vi "Injection Command Plot.vi"(6 "Plot Selector (T=TMP, F=EPT)":bool, 9 "System":T6={"Battery [V]"=13.7, "Engine Speed [RPM]"=1000.0, "Rotations"=1, "Injector Configuration"={"Resistance [Ohm]"=1.0, "Inductance [Henery]"=0.001, "Capacitance [Farad]"=5e-06}, "Description"=""} {"Injector Configuration"."Capacitance [Farad]" format="%#_6p"; "Injector Configuration"."Inductance [Henery]" format="%#_6p"; "Injector Configuration"."Resistance [Ohm]" format="%#_6p"; "Rotations" min=1 max=2; "Engine Speed [RPM]" min=500 max=50000; "Battery [V]" min=6 max=48}, 10 "Injection Command":T1={"Mode"=enum."Off", "Digital Input"=enum."Unused", "Default Profile Index"=0, "Cal Freq [Hz]"=0.0, "Cal Duration [s]"=0.0, "Cal Increment [s]"=0.0, "Cal Pulses"=0, "TMP Command Sequence"=[{"Duration [s]"=0.0, "Level"=FALSE, "Run/Stop"=FALSE, "Profile Index"=0}, {"Duration [s]"=0.0, "Level"=FALSE, "Run/Stop"=FALSE, "Profile Index"=0}, {"Duration [s]"=0.0, "Level"=FALSE, "Run/Stop"=FALSE, "Profile Index"=0}, {"Duration [s]"=0.0, "Level"=FALSE, "Run/Stop"=FALSE, "Profile Index"=0}, {"Duration [s]"=0.0, "Level"=FALSE, "Run/Stop"=FALSE, "Profile Index"=0}, {"Duration [s]"=0.0, "Level"=FALSE, "Run/Stop"=FALSE, "Profile Index"=0}, {"Duration [s]"=0.0, "Level"=FALSE, "Run/Stop"=FALSE, "Profile Index"=0}, {"Duration [s]"=0.0, "Level"=FALSE, "Run/Stop"=FALSE, "Profile Index"=0}], "EPT TDC Offset [CAD]"=0.0, "EPT Window Start [DBTDC]"=0.0, "EPT Window End [DBTDC]"=0.0, "EPT Angles"=[{"Enable"=FALSE, "Timing [DBTDC]"=0.0, "Duration [s]"=0.0, "Profile Index"=0}, {"Enable"=FALSE, "Timing [DBTDC]"=0.0, "Duration [s]"=0.0, "Profile Index"=0}, {"Enable"=FALSE, "Timing [DBTDC]"=0.0, "Duration [s]"=0.0, "Profile Index"=0}, {"Enable"=FALSE, "Timing [DBTDC]"=0.0, "Duration [s]"=0.0, "Profile Index"=0}, {"Enable"=FALSE, "Timing [DBTDC]"=0.0, "Duration [s]"=0.0, "Profile Index"=0}, {"Enable"=FALSE, "Timing [DBTDC]"=0.0, "Duration [s]"=0.0, "Profile Index"=0}, {"Enable"=FALSE, "Timing [DBTDC]"=0.0, "Duration [s]"=0.0, "Profile Index"=0}, {"Enable"=FALSE, "Timing [DBTDC]"=0.0, "Duration [s]"=0.0, "Profile Index"=0}], "EPT Skip Fire"=FALSE, "EPT Skip Index"=0, "EPT Precharge Duration [s]"=0.0, "EPT Precharge Profile Index"=0} {"EPT Precharge Profile Index" max=15; "EPT Precharge Duration [s]" min=0 format="%#_4p"; "Default Profile Index" max=15; "Cal Increment [s]" format="%#_3p"; "TMP Command Sequence"."Profile Index" max=7; "TMP Command Sequence"."Duration [s]" min=0 max=100 format="%#_3p"; "Cal Pulses" max=511; "EPT Skip Index" max=7; "EPT Angles"."Profile Index" max=7; "EPT Angles"."Duration [s]" min=0 max=100 format="%#_3p"; "Cal Duration [s]" format="%#_3p"; "Cal Freq [Hz]" format="%#_3p"}) -> (2 "Plot":cluster{"Array":sgl[], "Array":sgl[]}[](array[cluster]))   [LabVIEW 2016, in "DCM System Explorer.lvlib"]
uses:
  DCM System Explorer.lvlib
  <vilib>/Powertrain Controls/Device Drivers/DCM/Rev0/UI/System Configuration.ctl
  <vilib>/Powertrain Controls/Device Drivers/DCM/Rev0/UI/Injector Configuration.ctl
  <vilib>/Powertrain Controls/Device Drivers/DCM/DI/RT/Command.ctl
  <vilib>/Powertrain Controls/Device Drivers/DCM/DI/FPGA/Mode.ctl
  <vilib>/Powertrain Controls/Device Drivers/DCM/Rev0/FPGA/Digital Channel.ctl
  <vilib>/Powertrain Controls/Device Drivers/DCM/DI/RT/Command Sequence.ctl
  <vilib>/Powertrain Controls/Device Drivers/DCM/DI/RT/Angle Control.ctl
  <vilib>/Powertrain Controls/Device Drivers/DCM/Rev0/UI/DCM - UI.lvlib
  <vilib>/Powertrain Controls/Device Drivers/DCM/DI/FPGA/DCM - FPGA - DI.lvlib
  <vilib>/Powertrain Controls/Device Drivers/DCM/Rev0/FPGA/DCM - FPGA.lvlib
  <vilib>/Powertrain Controls/Device Drivers/DCM/DI/RT/DCM - RT - DI.lvlib
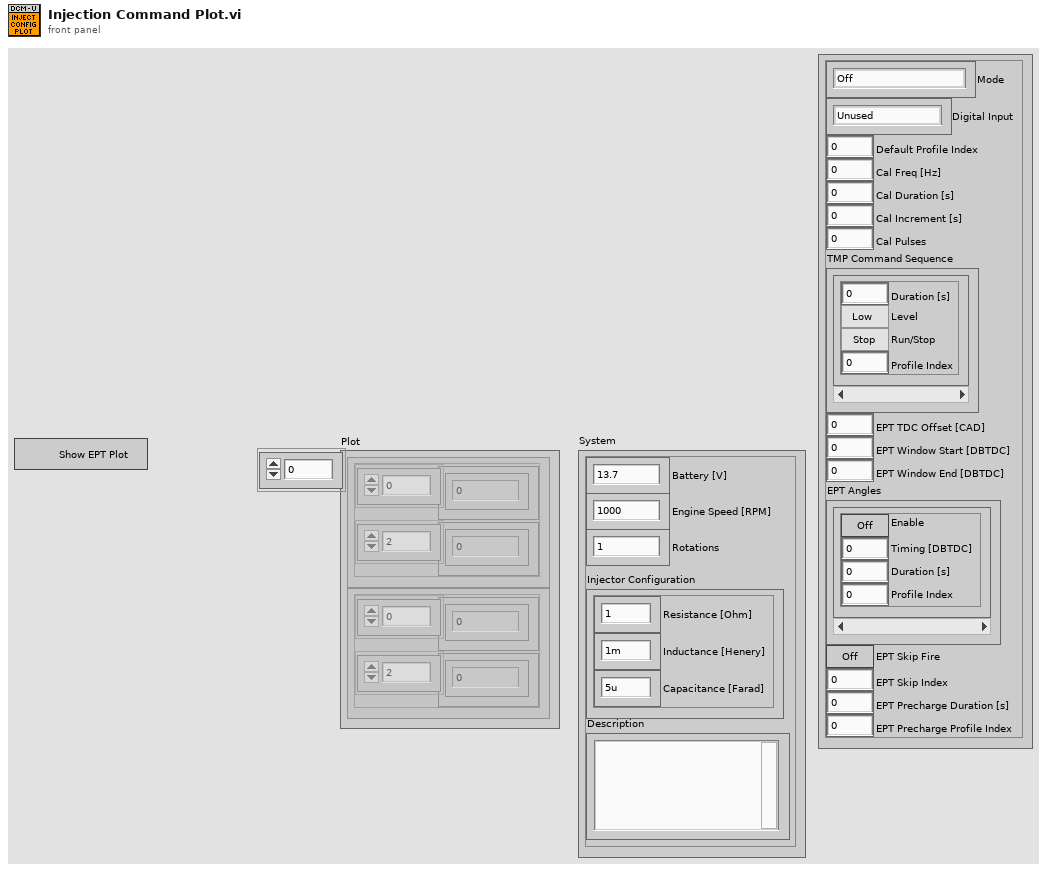
[diagram p1: front panel]
types:
  T1 = typedef "DCM - RT - DI.lvlib/Command.ctl" = cluster{"Mode":T2, "Digital Input":T3, "Default Profile Index":u8, "Cal Freq [Hz]":sgl, "Cal Duration [s]":sgl, "Cal Increment [s]":sgl, "Cal Pulses":u16, "TMP Command Sequence":T4[], "EPT TDC Offset [CAD]":sgl, "EPT Window Start [DBTDC]":sgl, "EPT Window End [DBTDC]":sgl, "EPT Angles":T5[], "EPT Skip Fire":bool, "EPT Skip Index":u8, "EPT Precharge Duration [s]":sgl, "EPT Precharge Profile Index":u8}
  T2 = typedef "DCM - FPGA - DI.lvlib/Mode.ctl" = enum8{"Off", "Direct", "Calibration", "Triggered Multi-Pulse", "Engine Position Tracking"}
  T3 = typedef "DCM - FPGA.lvlib/Digital Channel.ctl" = enum8{"Unused", "User OS", "Diff IO 1", "Diff IO 2", "Diff IO 3", "Diff IO 4", "Diff IO 5", "Diff IO 6", "Diff IO 7", "Diff IO 8", "Aux 1", "Aux 2", "Aux 3", "Aux 4", "Aux 5", "Aux 6", "Aux 7", "Aux 8", "Aux 9", "Aux 10", "Aux 11", "Aux 12", "Aux 13", "Aux 14", "Aux 15", "Aux 16"}
  T4 = typedef "DCM - RT - DI.lvlib/Command Sequence.ctl" = cluster{"Duration [s]":sgl, "Level":bool, "Run/Stop":bool, "Profile Index":u8}
  T5 = typedef "DCM - RT - DI.lvlib/Angle Control.ctl" = cluster{"Enable":bool, "Timing [DBTDC]":sgl, "Duration [s]":sgl, "Profile Index":u8}
  T6 = typedef "DCM - UI.lvlib/System Configuration.ctl" = cluster{"Battery [V]":sgl, "Engine Speed [RPM]":sgl, "Rotations":u8, "Injector Configuration":T7, "Description":string}
  T7 = typedef "DCM - UI.lvlib/Injector Configuration.ctl" = cluster{"Resistance [Ohm]":sgl, "Inductance [Henery]":sgl, "Capacitance [Farad]":sgl}
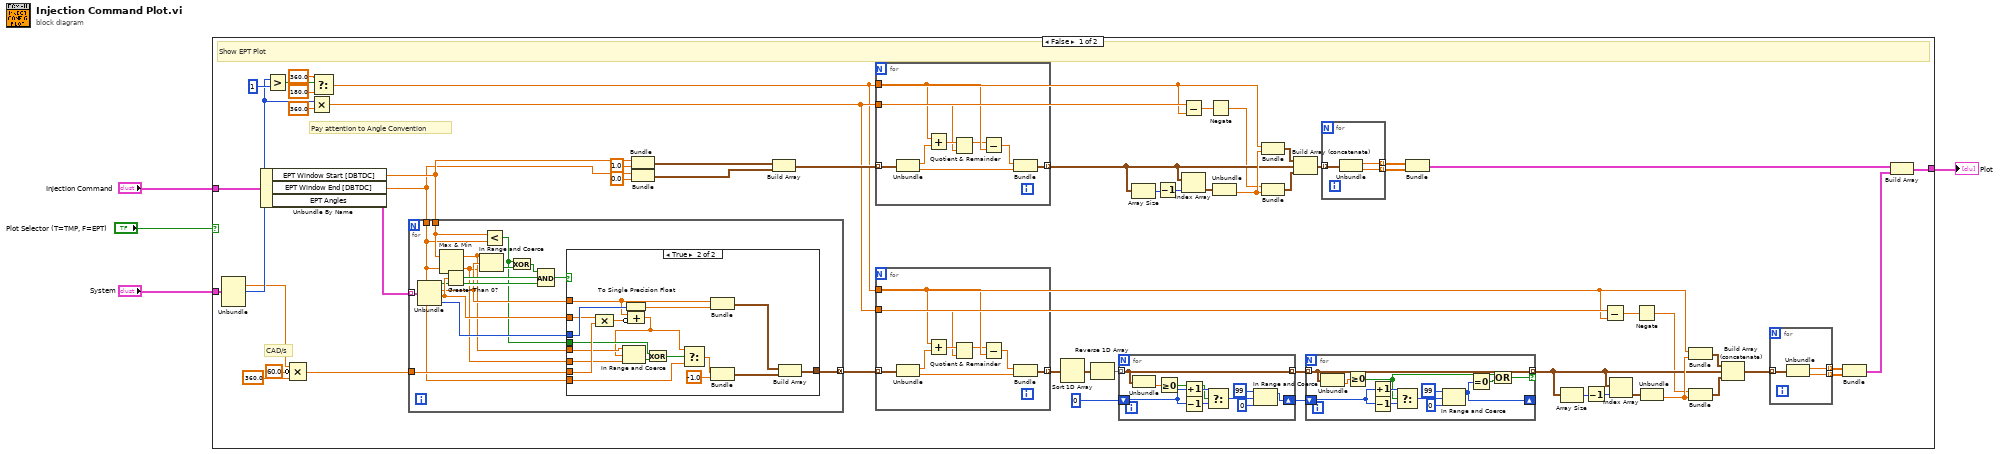
[diagram p0: block diagram]
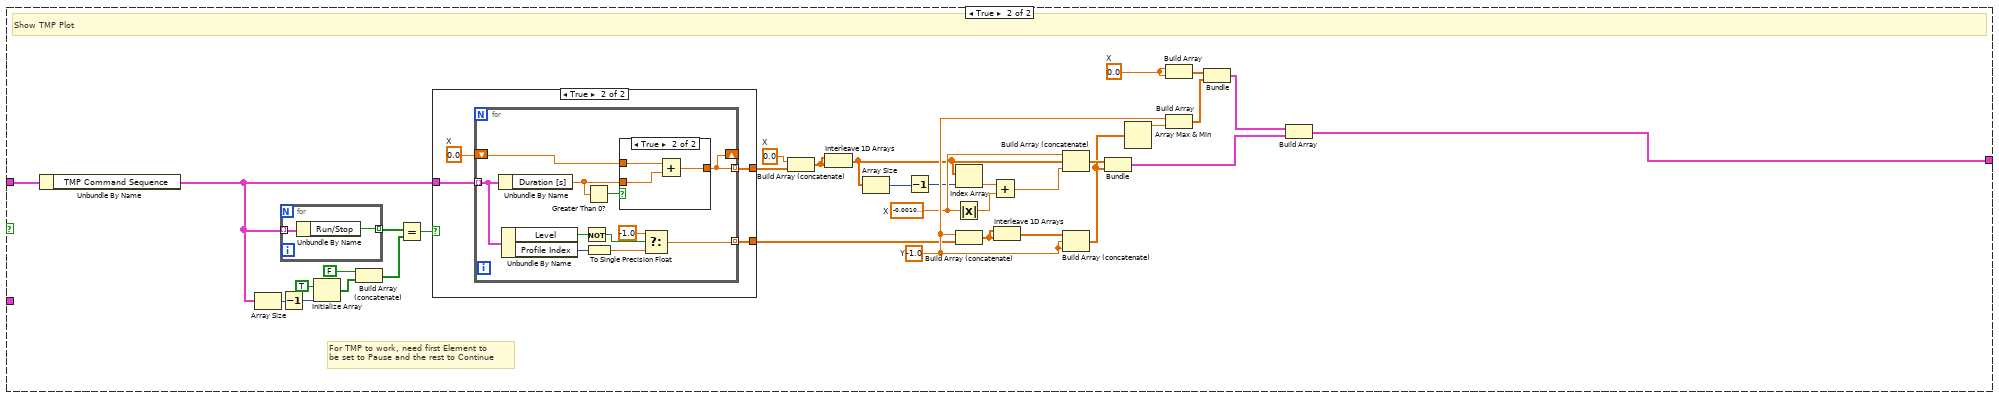
[diagram p3: hidden frame]
diagram:
  n1 = case shown="False" "Plot Selector (T=TMP, F=EPT)" {
    tunnel: "System" -> [w36 _]
    tunnel: [w25 w143] -> w1
    tunnel: "Injection Command" -> [w19 w145]
    frame False {
      # "Pay attention to Angle Convention"
      # "CAD/s"
      # "Show EPT Plot"
      n2 = Unbundle(w36) -> ("Engine Speed [RPM]"=w34:sgl, "Rotations"=w35:u8)  [unwired: 3 out]
      n3 = Unbundle By Name(w19) -> ("EPT Window Start [DBTDC]"=w17:sgl, "EPT Window End [DBTDC]"=w16:sgl, "EPT Angles"=w18:T5[])
      n4 = Greater?(x=w35, y=u8 1) -> (0:w56:bool)
      n5 = Compound Arithmetic op=MULTIPLY(w34, invert sgl 60.0 ("value"), sgl 360.0 ("value")) -> (w58:sgl)
      n6 = Multiply(x=w35, y=sgl 360.0) -> (x*y=w39:sgl)
      n7 = Select(t=sgl 360.0 ("y"), s=w56, f=sgl 180.0 ("y")) -> (s? t:f=w8:sgl)
      n8 = for {
        tunnel: [w76] -> w37 mode=concatenating
        tunnel: w58 -> [w75]
        tunnel: w18 -> [w74] mode=indexing
        tunnel: w17 -> [w64]
        tunnel: w16 -> [w61]
        n9 = Unbundle(w74) -> ("Enable"=w70:bool, "Timing [DBTDC]"=w67:sgl, "Duration [s]"=w72:sgl, "Profile Index"=w73:u8)
        n10 = Max & Min(x=w64, y=w61) -> (max(x,y)=w63:sgl, min(x,y)=w62:sgl)
        n11 = Greater Than 0?(x=w72) -> (x > 0?=w71:bool)
        n12 = In Range and Coerce(upper limit=w63, x=w67, lower limit=w62) -> (In Range?=w66:bool)  [unwired: 1 out]
        n13 = Less?(x=w64, y=w61) -> (x < y?=w65:bool)
        n14 = Exclusive Or(1:w66, 2:w65) -> (0:w68:bool)
        n15 = Compound Arithmetic op=AND(w68, w71, w70) -> (w69:bool)
        n16 = case shown="True" w69 {
          tunnel: [_ w94] -> w76
          tunnel: w67 -> [_ w87]
          tunnel: w72 -> [_ w89]
          tunnel: w73 -> [_ w93]
          tunnel: w75 -> [_ w85]
          tunnel: w65 -> [_ w83]
          tunnel: w62 -> [_ w82]
          tunnel: w63 -> [_ w81]
          tunnel: w61 -> [_ w78]
          frame False {
          }
          frame True {
            n17 = Compound Arithmetic op=MULTIPLY(w89, w85) -> (w90:sgl)
            n18 = To Single Precision Float(number=w93) -> (single precision float=w92:sgl)
            n19 = Compound Arithmetic op=ADD(w87, invert w90) -> (w79:sgl)
            n20 = In Range and Coerce(upper limit=w81, x=w79, lower limit=w82) -> (In Range?=w84:bool)  [unwired: 1 out]
            n21 = Exclusive Or(1:w84, 2:w83) -> (0:w80:bool)
            n22 = Select(t=w79, s=w80, f=w78) -> (s? t:f=w77:sgl)
            n23 = Bundle("Timing [DBTDC]"=w87, w92) -> (w86:cluster{"Timing [DBTDC]":sgl, sgl})  [unwired: 1 in]
            n24 = Bundle("EPT Window End [DBTDC]"=w77, sgl -1.0) -> (w88:cluster{"EPT Window End [DBTDC]":sgl, sgl})  [unwired: 1 in]
            n25 = Build Array(w86, w88) -> (w94:cluster{"EPT Window End [DBTDC]":sgl, sgl}[])
          }
        }
      }
      n26 = Bundle("EPT Window Start [DBTDC]"=w17, "y"=sgl 1.0) -> (w21:cluster{"EPT Window Start [DBTDC]":sgl, "y":sgl})  [unwired: 1 in]
      n27 = Bundle("EPT Window End [DBTDC]"=w16, "y"=sgl 0.0) -> (w20:cluster{"EPT Window End [DBTDC]":sgl, "y":sgl})  [unwired: 1 in]
      n28 = Build Array(w21, w20) -> (w52:cluster{"EPT Window End [DBTDC]":sgl, "y":sgl}[])
      n29 = for {
        tunnel: w52 -> [w140] mode=indexing
        tunnel: w8 -> [w135]
        tunnel: w39 -> [w136]
        tunnel: [w134] -> w12 mode=indexing
        n30 = Unbundle(w140) -> ("EPT Window End [DBTDC]"=w138:sgl, "y"=w139:sgl)
        n31 = Add(x=w135, y=w138) -> (x+y=w137:sgl)
        n32 = Quotient & Remainder(x=w137, y=w136) -> (x-y*floor(x/y)=w133:sgl)  [unwired: 1 out]
        n33 = Subtract(x=w133, y=w135) -> (x-y=w132:sgl)
        n34 = Bundle(w132, "y"=w139) -> (w134:cluster{sgl, "y":sgl})  [unwired: 1 in]
      }
      n35 = for {
        tunnel: w37 -> [w128] mode=indexing
        tunnel: w8 -> [w123]
        tunnel: w39 -> [w124]
        tunnel: [w121] -> w13 mode=indexing
        n36 = Unbundle(w128) -> ("EPT Window End [DBTDC]"=w126:sgl, w127:sgl)
        n37 = Add(x=w123, y=w126) -> (x+y=w125:sgl)
        n38 = Quotient & Remainder(x=w125, y=w124) -> (x-y*floor(x/y)=w120:sgl)  [unwired: 1 out]
        n39 = Subtract(x=w120, y=w123) -> (x-y=w122:sgl)
        n40 = Bundle(w122, w127) -> (w121:cluster{sgl, sgl})  [unwired: 1 in]
      }
      n41 = Sort 1D Array(array=w13) -> (sorted array=w6:cluster{sgl, sgl}[])
      n42 = Reverse 1D Array(array=w6) -> (reversed array=w5:cluster{sgl, sgl}[])
      n43 = for {
        tunnel: w5 -> [w100] mode=indexing
        tunnel: [w100] -> w28 mode=indexing
        shift-right: [w96] -> w26
        shift-left: 0 -> [w103]
        n44 = Unbundle(w100) -> (w104:sgl)  [unwired: 1 out]
        n45 = Greater Or Equal To 0?(x=w104) -> (x >= 0?=w95:bool)
        n46 = Increment(x=w103) -> (x+1=w101:i32)
        n47 = Decrement(x=w103) -> (x-1=w102:i32)
        n48 = Select(t=w101, s=w95, f=w102) -> (s? t:f=w99:i32)
        n49 = In Range and Coerce(upper limit=99, x=w99, lower limit=0) -> (coerced(x)=w96:i32)  [unwired: 1 out]
      }
      n50 = Array Size(array=w12) -> (size(s)=w31:i32)
      n51 = Decrement(x=w31) -> (x-1=w30:i32)
      n52 = Subtract(x=w39, y=w8) -> (x-y=w11:sgl)
      n53 = Index Array(array=w12, index=w30) -> (element=w47:cluster{sgl, "y":sgl})
      n54 = Negate(x=w11) -> (-x=w7:sgl)
      n55 = Unbundle(w47) -> ("y"=w46:sgl)  [unwired: 1 out]
      n56 = Bundle("y"=w8, "y"=w46) -> (w50:cluster{"y":sgl, "y":sgl})  [unwired: 1 in]
      n57 = Bundle(w7, "y"=w46) -> (w49:cluster{sgl, "y":sgl})  [unwired: 1 in]
      n58 = Build Array (concatenate)(w50, w12, w49) -> (w48:cluster{"y":sgl, "y":sgl}[])
      n59 = for {
        tunnel: w28 -> [w112] mode=indexing
        tunnel: [w112] -> w24 mode=indexing if=w105
        shift-right: [w108] -> _
        shift-left: w26 -> [w115]
        n60 = Unbundle(w112) -> (w116:sgl)  [unwired: 1 out]
        n61 = Greater Or Equal To 0?(x=w116) -> (x >= 0?=w106:bool)
        n62 = Increment(x=w115) -> (x+1=w113:i32)
        n63 = Decrement(x=w115) -> (x-1=w114:i32)
        n64 = Select(t=w113, s=w106, f=w114) -> (s? t:f=w111:i32)
        n65 = In Range and Coerce(upper limit=99, x=w111, lower limit=0) -> (coerced(x)=w108:i32)  [unwired: 1 out]
        n66 = Equal To 0?(x=w108) -> (x = 0?=w107:bool)
        n67 = Compound Arithmetic op=OR(w106, w107) -> (w105:bool)
      }
      n68 = for {
        tunnel: w48 -> [w131] mode=indexing
        tunnel: [w130] -> w10 mode=indexing
        tunnel: [w129] -> w9 mode=indexing
        n69 = Unbundle(w131) -> ("y"=w130:sgl, "y"=w129:sgl)
      }
      n70 = Bundle(w10, w9) -> (w51:cluster{sgl[], sgl[]})  [unwired: 1 in]
      n71 = Array Size(array=w24) -> (size(s)=w33:i32)
      n72 = Decrement(x=w33) -> (x-1=w32:i32)
      n73 = Subtract(x=w39, y=w8) -> (x-y=w15:sgl)
      n74 = Index Array(array=w24, index=w32) -> (element=w44:cluster{sgl, sgl})
      n75 = Negate(x=w15) -> (-x=w14:sgl)
      n76 = Unbundle(w44) -> (w45:sgl)  [unwired: 1 out]
      n77 = Bundle("y"=w8, w45) -> (w42:cluster{"y":sgl, sgl})  [unwired: 1 in]
      n78 = Bundle(w14, w45) -> (w43:cluster{sgl, sgl})  [unwired: 1 in]
      n79 = Build Array (concatenate)(w42, w24, w43) -> (w29:cluster{"y":sgl, sgl}[])
      n80 = for {
        tunnel: w29 -> [w119] mode=indexing
        tunnel: [w118] -> w40 mode=indexing
        tunnel: [w117] -> w41 mode=indexing
        n81 = Unbundle(w119) -> ("y"=w118:sgl, w117:sgl)
      }
      n82 = Bundle(w40, w41) -> (w38:cluster{sgl[], sgl[]})  [unwired: 1 in]
      n83 = Build Array(w51, w38) -> (w25:cluster{sgl[], sgl[]}[])
    }
    frame True {
      w141 = sgl 0.0  # X
      w151 = sgl 0.0  # X
      w164 = sgl -1.0  # Y
      w163 = sgl -0.001  # X
      # "For TMP to work, need first Element to\nbe set to Pause and the rest to Continue"
      # "Show TMP Plot"
      n84 = Unbundle By Name(w145) -> ("TMP Command Sequence"=w144:T4[])
      n85 = Array Size(array=w144) -> (size(s)=w172:i32)
      n86 = for {
        tunnel: w144 -> [w194] mode=indexing
        tunnel: [w193] -> w166 mode=indexing
        n87 = Unbundle By Name(w194) -> ("Run/Stop"=w193:bool)
      }
      n88 = Decrement(x=w172) -> (x-1=w173:i32)
      n89 = Initialize Array(TRUE, w173) -> (w169:bool[])
      n90 = Build Array (concatenate)(FALSE, w169) -> (w170:bool[])
      n91 = Equal?(x=w166, y=w170) -> (x = y?=w171:bool)
      n92 = case shown="True" w171 {
        tunnel: [_ w176] -> w146
        tunnel: [_ w175] -> w147
        tunnel: w144 -> [_ w174]
        frame False {
        }
        frame True {
          w177 = sgl 0.0  # X
          n93 = for {
            tunnel: w174 -> [w186] mode=indexing
            shift-right: [w179] -> _
            shift-left: w177 -> [w180]
            tunnel: [w179] -> w176 mode=indexing
            tunnel: [w181] -> w175 mode=indexing
            n94 = Unbundle By Name(w186) -> ("Duration [s]"=w187:sgl)
            n95 = Unbundle By Name(w186) -> ("Level"=w184:bool, "Profile Index"=w185:u8)
            n96 = Not(x=w184) -> (.not. x?=w178:bool)
            n97 = Greater Than 0?(x=w187) -> (x > 0?=w188:bool)
            n98 = To Single Precision Float(number=w185) -> (single precision float=w183:sgl)
            n99 = case shown="True" w188 {
              tunnel: w187 -> [_ w192]
              tunnel: w180 -> [w189 w191]
              tunnel: [w189 w190] -> w179
              frame False {
              }
              frame True {
                n100 = Add(x=w191, y=w192) -> (x+y=w190:sgl)
              }
            }
            n101 = Select(t=sgl -1.0 ("Y"), s=w178, f=w183) -> (s? t:f=w181:sgl)
          }
        }
      }
      n102 = Build Array (concatenate)(w151, w146) -> (w150:sgl[])
      n103 = Interleave 1D Arrays(w150, w150) -> (w156:sgl[])
      n104 = Array Size(array=w156) -> (size(s)=w153:i32)
      n105 = Decrement(x=w153) -> (x-1=w154:i32)
      n106 = Absolute Value(x=w163) -> (abs(x)=w157:sgl)
      n107 = Index Array(array=w156, index=w154) -> (element=w155:sgl)
      n108 = Build Array (concatenate)(w164, w147) -> (w148:sgl[])
      n109 = Add(x=w155, y=w157) -> (x+y=w158:sgl)
      n110 = Interleave 1D Arrays(w148, w148) -> (w152:sgl[])
      n111 = Build Array (concatenate)(w163, w156, w158) -> (w149:sgl[])
      n112 = Build Array (concatenate)(w152, w164, w164) -> (w142:sgl[])
      n113 = Bundle(w149, w142) -> (w159:cluster{sgl[], sgl[]})  [unwired: 1 in]
      n114 = Array Max & Min(array=w142) -> (max value=w165:sgl)  [unwired: 3 out]
      n115 = Build Array(w141, w141) -> (w160:sgl[])
      n116 = Build Array(w164, w165) -> (w161:sgl[])
      n117 = Bundle(w160, w161) -> (w162:cluster{sgl[], sgl[]})  [unwired: 1 in]
      n118 = Build Array(w162, w159) -> (w143:cluster{sgl[], sgl[]}[])
    }
  }
  "Plot" <- w1
